vi "Get Sheet.vi"(8 "error in":errorcluster, 10 "SheetName":string, 11 "SpreadsheetDoc in":refnum<k24>) -> (0 "error out":errorcluster, 1 "Sheet Index":i32, 2 "Sheet":refnum<k24>, 3 "SpreadsheetDoc out":refnum<k24>)   [LabVIEW 2019, in "Open Xml.lvlib"]
doc: "Returns first sheet on empty Sheet Name"
uses:
  Open Xml.lvlib
  D:/git/Open-Xml-LabVIEW/Source/DocumentFormat.OpenXml.dll
  DocumentFormat.OpenXml.dll
  D:/git/Open-Xml-LabVIEW/Source/DocumentFormat.OpenXml.Framework.dll
  DocumentFormat.OpenXml.Framework.dll
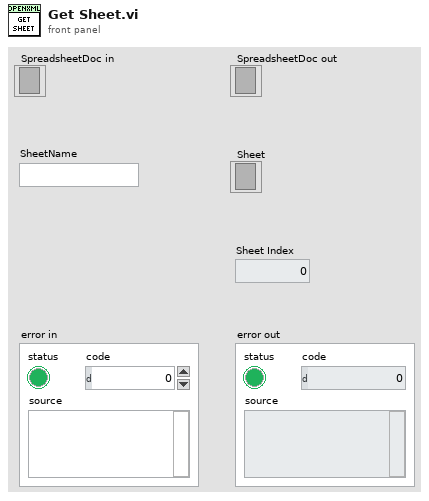
[diagram p1: front panel]
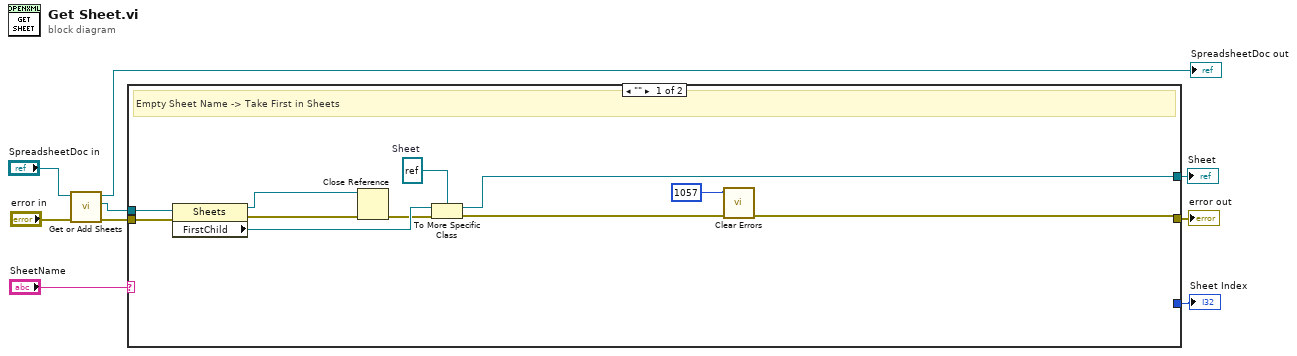
[diagram p0: block diagram]
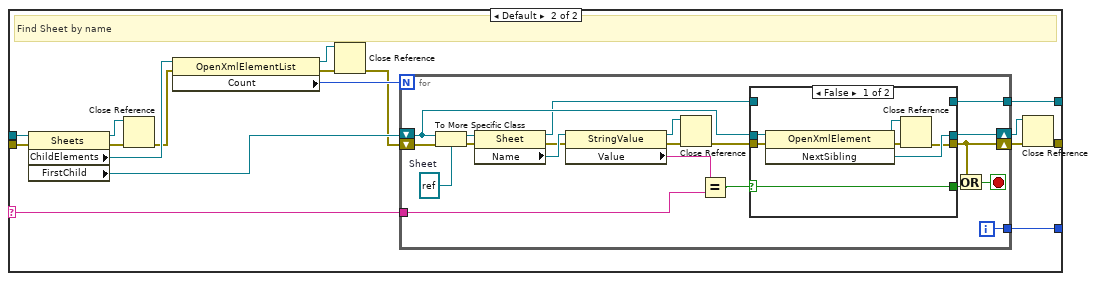
[diagram p2: hidden frame]
diagram:
  n1 = call "Get or Add Sheets.vi"("error in"="error in", "SpreadsheetDoc in"="SpreadsheetDoc in") -> ("error out"=w6:errorcluster, "Sheets"=w7:refnum<k24>, "SpreadsheetDoc out"=→"SpreadsheetDoc out":refnum<k24>)  [unwired: 7 in]
  n2 = case shown="\"\"" "SheetName" {
    selector: "SheetName" -> [_ w31]
    tunnel: w7 -> [w19 w33]
    tunnel: w6 -> [w20 w32]
    tunnel: [w12 w29] -> w3
    tunnel: [w11 w27] -> w2
    tunnel: [_ w21] -> w1
    frame "" {
      w17 = refnum<k24> refnum  # Sheet
      # "Empty Sheet Name -> Take First in Sheets"
      n3 = property class="Sheets"(reference=w19, error in=w20) -> (reference out=w14:refnum<k24>, error out=w18:errorcluster, "FirstChild"=w16:refnum<k24>)
      n4 = Close Reference(reference=w14, error in (no error)=w18) -> (error out=w15:errorcluster)
      n5 = To More Specific Class(target class=w17, reference=w16, error in=w15) -> (specific class reference=w12:refnum<k24>, error out=w13:errorcluster)
      n6 = call <vilib>:"Clear Errors.vi"("error in (no error)"=w13, "specific error code to clear (0: all)"=1057) -> ("error out"=w11:errorcluster)  [unwired: 4 in, 1 out]
    }
    frame Default {
      # "Find Sheet by name"
      n7 = property class="Sheets"(reference=w33, error in=w32) -> (reference out=w30:refnum<k24>, error out=w37:errorcluster, "ChildElements"=w35:refnum<k24>, "FirstChild"=w36:refnum<k24>)
      n8 = Close Reference(reference=w30, error in (no error)=w37) -> (error out=w25:errorcluster)
      n9 = property class="OpenXmlElementList"(reference=w35, error in=w25) -> (reference out=w22:refnum<k24>, error out=w24:errorcluster, "Count"=w34:i32)
      n10 = Close Reference(reference=w22, error in (no error)=w24) -> (error out=w23:errorcluster)
      n11 = for {
        N: w34 -> [_]
        shift-right: [w50] -> w26
        shift-left: w36 -> [w53]
        tunnel: w31 -> [w51]
        tunnel: [w44] -> w29
        shift-right: [w45] -> w28
        shift-left: w23 -> [w56]
        tunnel: [w38] -> w21
        i -> [w38]
        stop <- w46 stop-if-true
        w57 = refnum<k24> refnum  # Sheet
        n12 = To More Specific Class(target class=w57, reference=w53, error in=w56) -> (specific class reference=w52:refnum<k24>, error out=w55:errorcluster)
        n13 = property class="Sheet"(reference=w52, error in=w55) -> (reference out=w49:refnum<k24>, error out=w41:errorcluster, "Name"=w43:refnum<k24>)
        n14 = property class="StringValue"(reference=w43, error in=w41) -> (reference out=w39:refnum<k24>, error out=w40:errorcluster, "Value"=w42:string)
        n15 = Close Reference(reference=w39, error in (no error)=w40) -> (error out=w54:errorcluster)
        n16 = Equal?(x=w42, y=w51) -> (x = y?=w48:bool)
        n17 = case shown="False" w48 {
          selector: w48 -> [w61 w67]
          tunnel: w54 -> [w64 w66]
          tunnel: [w58 w66] -> w45
          tunnel: w53 -> [w63 _]
          tunnel: [w62 _] -> w50
          tunnel: w49 -> [_ w65]
          tunnel: [w61 w67] -> w47
          tunnel: [_ w65] -> w44
          frame False {
            n18 = invoke class="OpenXmlElement" method="NextSibling"(reference=w63, error in=w64) -> (reference out=w60:refnum<k24>, error out=w59:errorcluster, "NextSibling"=w62:refnum<k24>)  [unwired: 1 in]
            n19 = Close Reference(reference=w60, error in (no error)=w59) -> (error out=w58:errorcluster)
          }
          frame True {
          }
        }
        n20 = Or(x=w45, y=w47) -> (x .or. y?=w46:bool)
      }
      n21 = Close Reference(reference=w26, error in (no error)=w28) -> (error out=w27:errorcluster)
    }
  }
  "error out" <- w2
  "Sheet" <- w3
  "Sheet Index" <- w1
